vi "Read timeouts.vi"(8 "error in (no error)":errorcluster, 11 "TCP in":refnum<class "TCP.lvclass">) -> (0 "error out":errorcluster, 2 "timeouts":T1={"connect timeout"=60000, "write timeout"=10000, "read timeout"=10000}, 3 "TCP out":refnum<class "TCP.lvclass">)   [LabVIEW 2021, in "TCP.lvclass"]
uses:
  TCP.lvclass
  tcp timeouts.ctl
  TCP.lvclass/TCP.ctl
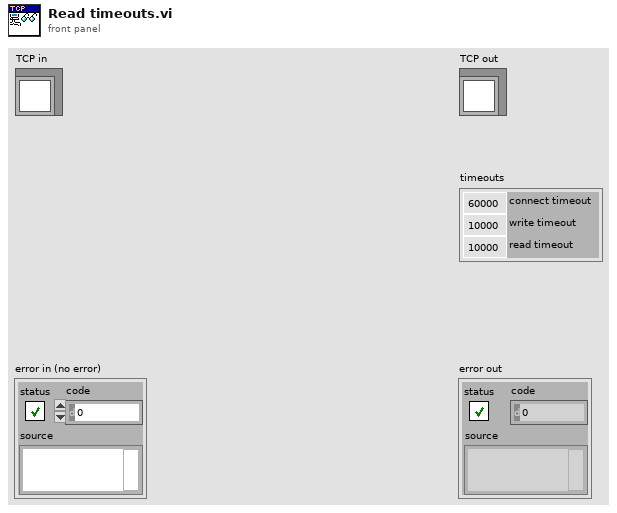
[diagram p1: front panel]
types:
  T1 = typedef "TCP.lvclass/tcp timeouts.ctl" = cluster{"connect timeout":i32, "write timeout":i32, "read timeout":i32}
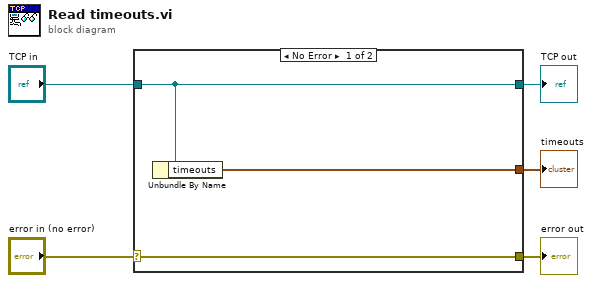
[diagram p0: block diagram]
diagram:
  n1 = case shown="No Error" "error in (no error)" {
    selector: "error in (no error)" -> [w8 w9]
    tunnel: [w8 w9] -> w4
    tunnel: [w7 w10] -> w2
    tunnel: "TCP in" -> [w7 w10]
    tunnel: [w6 _] -> w1
    frame No Error {
      n2 = Unbundle By Name(w7) -> ("timeouts"=w6:T1)
    }
    frame Error {
    }
  }
  "error out" <- w4
  "TCP out" <- w2
  "timeouts" <- w1
